vi "HexaboardCenterFinderLaserHoleAI.vi"() -> ()   [LabVIEW 2019]
uses:
  <vilib>/userDefined/High Color/IMAQdx.ctl
  <vilib>/Analysis/coordinate.llb/2D Cartesian Coordinate Rotation (Scalar).vi
  <vilib>/Utility/file.llb/Read Delimited Spreadsheet (DBL).vi
  Other Models/2010/Motion/AbortSingle.vi
  <vilib>/Analysis/NI_AALPro.lvlib
panel:
  out "error out":errorcluster
  out "CameraGcode":string
  out "Center_XYZU":string
  out "Image 2":T1(plugin-control)
  out "Image":T1(plugin-control)
  in  "YoffsetPos1":dbl=24.138
  in  "XoffsetPos1":dbl=6.964
  in  "ModuleName":string="T1"
  in  "StopJoyStick":bool
  out "CurrentImage":T1(plugin-control)
  in  "CoordFileIn":string="HB_LaserHoles.txt"
  out "UsedCoordinates":string
  in  "Position":enum16{"1", "2"}(ring)
  in  "Zone":enum16{"ZoneA", "ZoneB", "ZoneC", "ZoneD"}(ring)
  in  "InitialStepSize":dbl=0.05
  in  "AbortAutoFocus":bool
  in  "AutoFocus":bool=TRUE
  in  "VisibilityInCamera":enum16{"JoyStick", "AllVisible"}(ring)=enum."AllVisible"
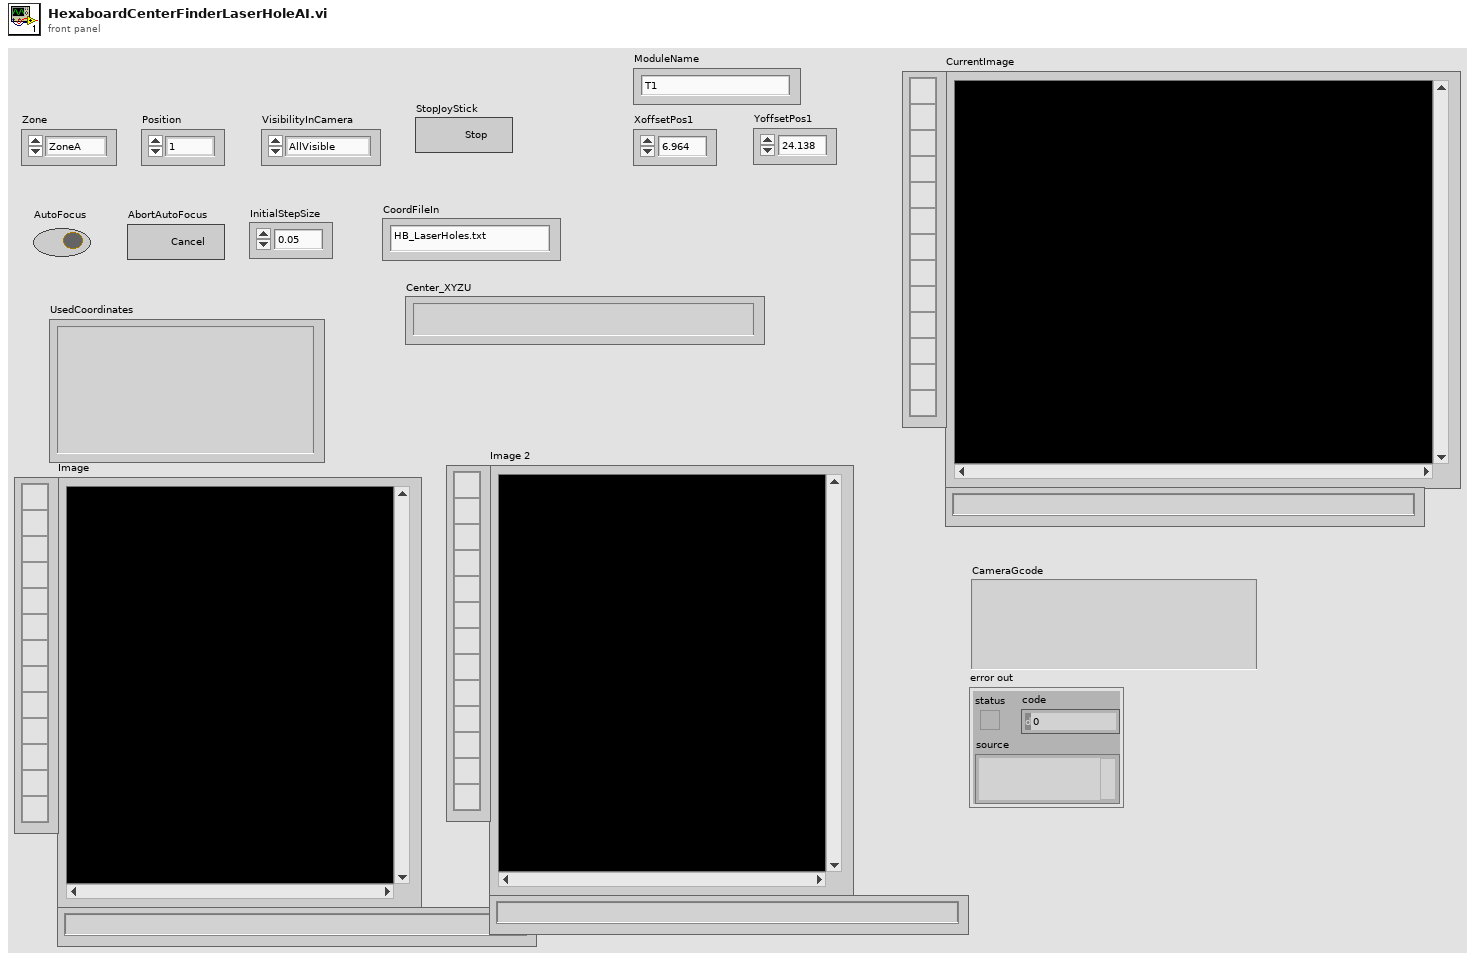
[diagram p1: front panel]
types:
  T1 = typedef "IMAQ Image.ctl" = refnum<image>
  T2 = typedef "Image Type" = u32
  T3 = typedef "IMAQdx.ctl" = refnum<k21>
  T4 = enum16{"Left Button", "Center Button", "Right Button", "Window Close"}
  T5 = enum16{"open", "replace", "create", "open or create", "replace or create", "replace or create with confirmation"}
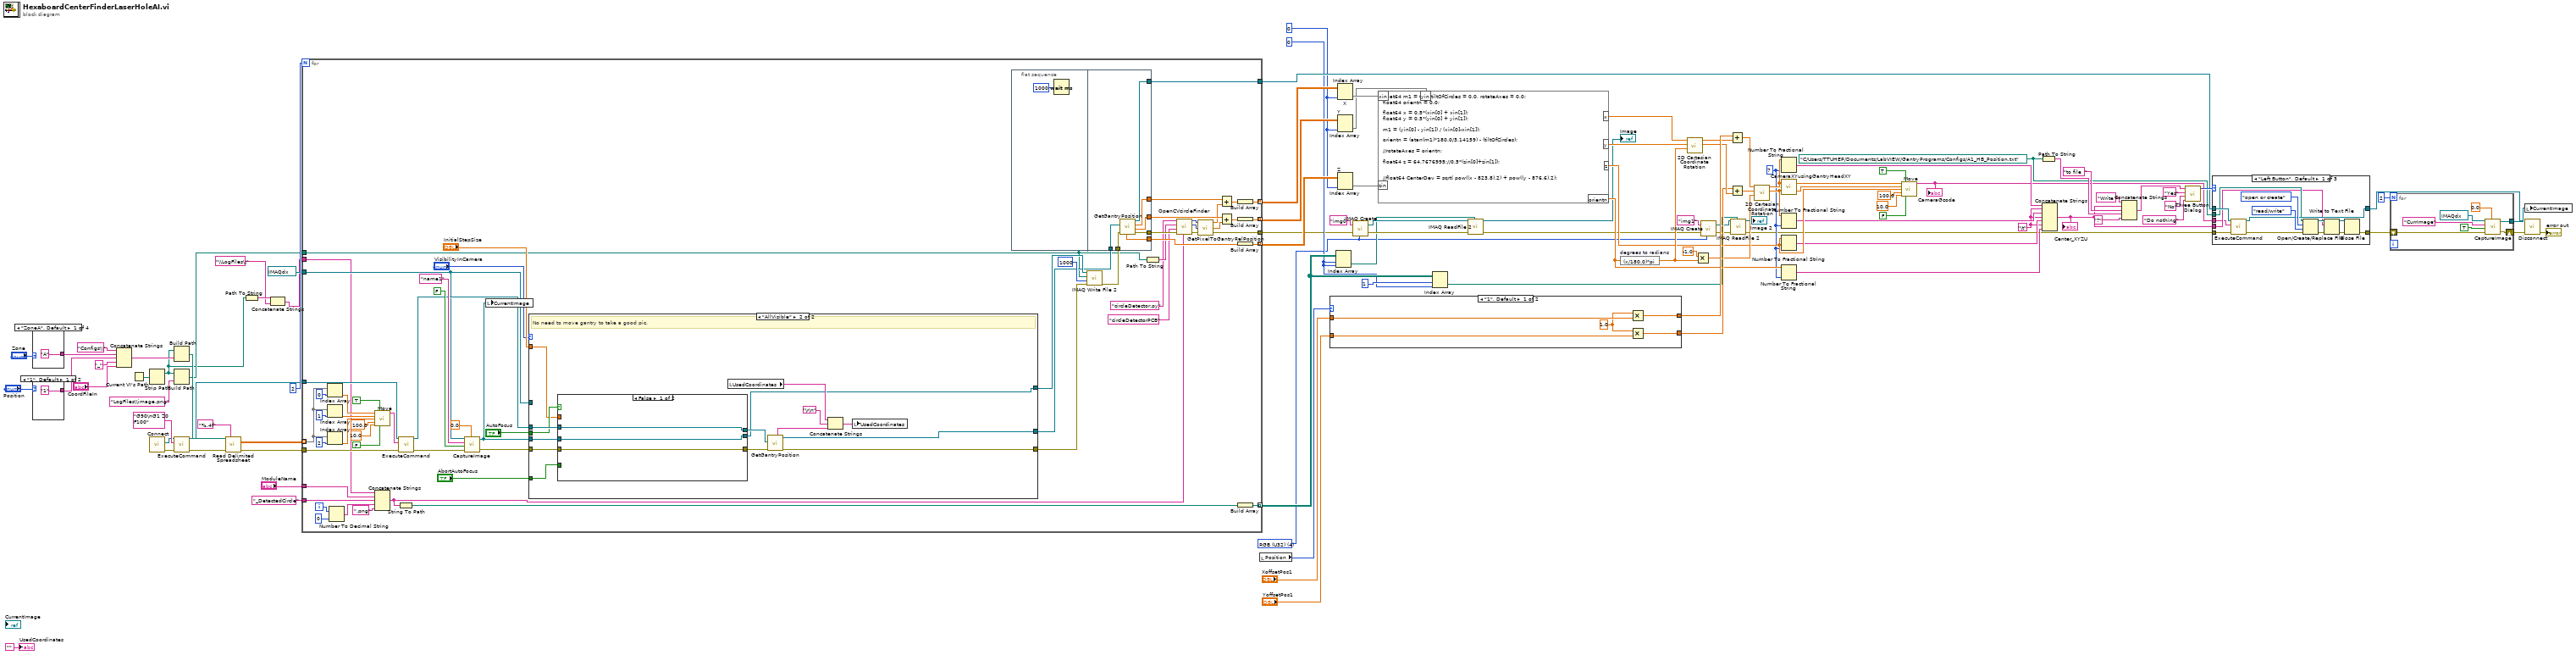
[diagram p0: block diagram]
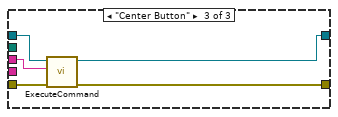
[diagram p3: hidden frame]
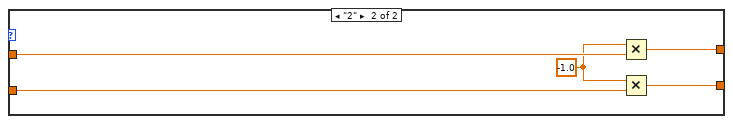
[diagram p4: hidden frame]
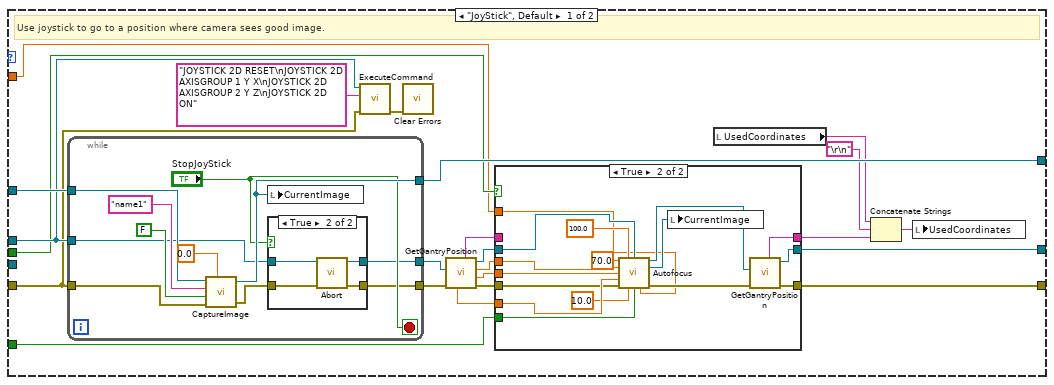
[diagram p5: hidden frame]
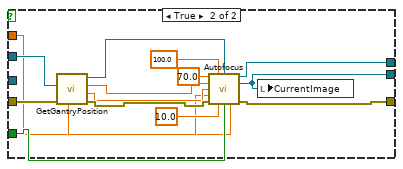
[diagram p8: hidden frame]
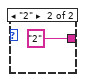
[diagram p9: hidden frame]
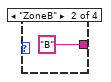
[diagram p10: hidden frame]
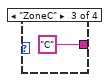
[diagram p11: hidden frame]
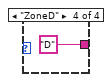
[diagram p12: hidden frame]
diagram:
  w14 = T2 4 items=["Grayscale (U8)", "Grayscale (I16)", "Grayscale (SGL)", "Complex (CSG)", "RGB (U32)", "HSL (U32)", "RGB (U64)", "Grayscale (U16)"] ("Image Type")
  w18 = 0 ("index")
  w44 = "\t"
  w45 = i16 7 ("precision (6)")
  w33 = path "C:/Users/TTUHEP/Documents/LabVIEW/GantryPrograms/Configs/A1_HB_Position.txt" ("OutFile")
  w24 = 0 ("disabled index (col)")
  n1 = case shown="\"ZoneA\", Default" "Zone" {
    tunnel: ["A" "B" "C" "D"] -> w99
    frame "ZoneA", Default {
    }
    frame "ZoneB" {
    }
    frame "ZoneC" {
    }
    frame "ZoneD" {
    }
  }
  n2 = case shown="\"1\", Default" "Position" {
    tunnel: ["1" "2"] -> w98
    frame "1", Default {
    }
    frame "2" {
    }
  }
  n3 = Concatenate Strings("Configs\\" ("string"), w99, w98, "_" ("string"), "CoordFileIn") -> (w93:string)
  n4 = Current VI's Path() -> (path=w96:path)
  n5 = Strip Path(path=w96) -> (stripped path=w4:path)  [unwired: 1 out]
  n6 = call "Connect.vi"() -> ("error out"=w90:errorcluster, "controller"=w91:refnum<k24>)  [unwired: 10 in]
  n7 = Build Path(base path=w4, name or relative path=w93) -> (appended path=w88:path)
  n8 = Build Path(base path=w4, name or relative path="LogFiles\\image.png") -> (appended path=w80:path)
  n9 = call "ExecuteCommand.vi"("error in (no error)"=w90, "Command Code"="G90\nG1 Z0 F100", "controller in"=w91) -> ("error out"=w87:errorcluster, "controller out"=w84:refnum<k24>)  [unwired: 6 in, 1 out]
  n10 = call-poly <vilib>:"Read Delimited Spreadsheet.vi"("file path (dialog if empty)"=w88, "format (%.3f)"="%.4f", "error in (no error)"=w87) -> ("all rows"=w86:dbl[][], "error out"=w83:errorcluster)  [unwired: 7 in, 4 out]
  n11 = Path To String(path=w4) -> (string=w3:string)
  n12 = Concatenate Strings(w3, "\\LogFiles\\") -> (w1:string)
  n13 = for {
    N: 2 -> [_]
    tunnel: w86 -> [w167] mode=indexing
    tunnel: w84 -> [w158]
    tunnel: w83 -> [w157]
    tunnel: T3 "cam1" ("Camera") -> [w149]
    tunnel: w80 -> [w116]
    tunnel: w1 -> [w137]
    tunnel: "ModuleName" -> [w136]
    tunnel: "_DetectedCircle" ("string") -> [w135]
    tunnel: [w129] -> w77 mode=indexing
    tunnel: [w128] -> w76 mode=indexing
    tunnel: [w126] -> w25 mode=indexing
    tunnel: [w125] -> w34
    tunnel: [w112] -> w8
    tunnel: [w111] -> w19 mode=indexing
    i -> [w134]
    n14 = Index Array(array=w167, index=0) -> (element=w166:dbl)
    n15 = Index Array(array=w167, index=1) -> (element=w165:dbl)
    n16 = Index Array(array=w167, index=2) -> (element=w164:dbl)
    n17 = Number To Decimal String(number=w134, width (-)=i16 0) -> (decimal integer string=w123:string)
    n18 = call "Move.vi"("X"=w166, "Absolute"=TRUE, "Y"=w165, "Z"=w164, "SpeedXY (mm/s)"=100.0, "SpeedZ (mm/s)"=10.0, "Move Z first"=FALSE) -> ("Position Gcode"=w159:string)  [unwired: 8 in]
    n19 = Concatenate Strings(w137, w136, w135, w123, ".png" ("string")) -> (w110:string)
    n20 = String To Path(string=w110) -> (path=w109:path)
    n21 = call "ExecuteCommand.vi"("error in (no error)"=w157, "Command Code"=w159, "controller in"=w158) -> ("error out"=w154:errorcluster, "controller out"=w150:refnum<k24>)  [unwired: 6 in, 1 out]
    n22 = call "CaptureImage.vi"("Camera"=w149, "Rotate (degrees)"=sgl 0.0, "ImageName"="name1", "Draw50MicroCircleAtCenter"=FALSE, "error in (no error)"=w154) -> ("Image"=w145:T1, "error out"=w148:errorcluster)  [unwired: 2 in]
    n23 = local write "CurrentImage"(w145) -> ()
    n24 = case shown="\"AllVisible\"" "VisibilityInCamera" {
      tunnel: w149 -> [w199 _]
      tunnel: w150 -> [w197 w250]
      tunnel: w148 -> [w195 w251]
      tunnel: [w198 w239] -> w143
      tunnel: [w182 w245] -> w140
      tunnel: [w183 w243] -> w142
      tunnel: "AbortAutoFocus" -> [w186 w248]
      tunnel: "AutoFocus" -> [w180 w249]
      tunnel: "InitialStepSize" -> [w179 w247]
      tunnel: w145 -> [_ w238]
      frame "JoyStick", Default {
        # "Use joystick to go to a position where camera sees good image."
        n25 = while {
          tunnel: w199 -> [w229]
          tunnel: [w226] -> w198
          tunnel: w197 -> [w225]
          tunnel: [w222] -> w193
          tunnel: [w221] -> w194
          tunnel: w195 -> [w220]
          stop <- "StopJoyStick" stop-if-true
          n26 = call "CaptureImage.vi"("Camera"=w229, "Rotate (degrees)"=sgl 0.0, "ImageName"="name1", "Draw50MicroCircleAtCenter"=FALSE, "error in (no error)"=w220) -> ("Image"=w226:T1, "error out"=w223:errorcluster)  [unwired: 2 in]
          n27 = local write "CurrentImage"(w226) -> ()
          n28 = case shown="True" "StopJoyStick" {
            tunnel: w225 -> [w232 w236]
            tunnel: w223 -> [w231 w235]
            tunnel: [w231 w234] -> w222
            tunnel: [w232 w233] -> w221
            frame False {
            }
            frame True {
              n29 = call-poly "Abort.vi"("error in (no error)"=w235, "controller in"=w236) -> ("error out"=w234:errorcluster, "controller out"=w233:refnum<k24>)  [unwired: 8 in]
            }
          }
        }
        n30 = call "ExecuteCommand.vi"("error in (no error)"=w195, "Command Code"="JOYSTICK 2D RESET\nJOYSTICK 2D AXISGROUP 1 Y X\nJOYSTICK 2D AXISGROUP 2 Y Z\nJOYSTICK 2D ON", "controller in"=w197) -> ("error out"=w196:errorcluster)  [unwired: 6 in, 2 out]
        n31 = call <vilib>:"Clear Errors.vi"("error in (no error)"=w196) -> ()  [unwired: 5 in, 2 out]
        n32 = call "GetGantryPosition.vi"("error in (no error)"=w193, "Controller In"=w194) -> ("error out"=w187:errorcluster, "Position Y"=w189:dbl, "Position X"=w190:dbl, "controller out"=w185:refnum<k24>, "Position_XYZ"=w181:string, "Position Z"=w188:dbl)  [unwired: 3 in, 1 out]
        n33 = case shown="True" w180 {
          tunnel: w190 -> [_ w219]
          tunnel: w189 -> [_ w218]
          tunnel: w188 -> [_ w217]
          tunnel: w187 -> [w203 w216]
          tunnel: w186 -> [_ w214]
          tunnel: w185 -> [w201 w213]
          tunnel: [w202 w209] -> w184
          tunnel: [w203 w208] -> w183
          tunnel: [w201 w207] -> w182
          tunnel: w181 -> [w202 _]
          tunnel: w179 -> [_ w205]
          frame False {
          }
          frame True {
            n34 = call "Autofocus.vi"("SafeMaxZ"=70.0, "SpeedXY (mm/s)"=100.0, "controller in"=w213, "X"=w219, "Y"=w218, "Z"=w217, "error in (no error)"=w216, "SpeedZ (mm/s)"=10.0, "AbortAutoFocus"=w214, "InitialStepSize"=w205) -> ("controller out"=w211:refnum<k24>, "Image"=w206:T1, "error out"=w210:errorcluster)  [unwired: 1 in, 2 out]
            n35 = local write "CurrentImage"(w206) -> ()
            n36 = call "GetGantryPosition.vi"("error in (no error)"=w210, "Controller In"=w211) -> ("error out"=w208:errorcluster, "controller out"=w207:refnum<k24>, "Position_XYZ"=w209:string)  [unwired: 3 in, 4 out]
          }
        }
        n37 = local read "UsedCoordinates"() -> (w191:string)
        n38 = Concatenate Strings(w191, "\r\n", w184) -> (w192:string)
        n39 = local write "UsedCoordinates"(w192) -> ()
      }
      frame "AllVisible" {
        # "No need to move gantry to take a good pic."
        n40 = case shown="False" w249 {
          tunnel: w248 -> [_ w268]
          tunnel: [w254 w265] -> w244
          tunnel: [w253 w266] -> w246
          tunnel: w251 -> [w254 w264]
          tunnel: w250 -> [w253 w263]
          tunnel: w247 -> [_ w257]
          tunnel: w238 -> [w252 _]
          tunnel: [w252 w256] -> w239
          frame False {
          }
          frame True {
            n41 = call "GetGantryPosition.vi"("error in (no error)"=w264, "Controller In"=w263) -> ("error out"=w262:errorcluster, "Position Y"=w261:dbl, "Position X"=w260:dbl, "controller out"=w259:refnum<k24>, "Position Z"=w258:dbl)  [unwired: 3 in, 2 out]
            n42 = call "Autofocus.vi"("SafeMaxZ"=70.0, "SpeedXY (mm/s)"=100.0, "controller in"=w259, "X"=w260, "Y"=w261, "Z"=w258, "error in (no error)"=w262, "SpeedZ (mm/s)"=10.0, "AbortAutoFocus"=w268, "InitialStepSize"=w257) -> ("controller out"=w266:refnum<k24>, "Image"=w256:T1, "error out"=w265:errorcluster)  [unwired: 1 in, 2 out]
            n43 = local write "CurrentImage"(w256) -> ()
          }
        }
        n44 = local read "UsedCoordinates"() -> (w241:string)
        n45 = call "GetGantryPosition.vi"("error in (no error)"=w244, "Controller In"=w246) -> ("error out"=w243:errorcluster, "controller out"=w245:refnum<k24>, "Position_XYZ"=w242:string)  [unwired: 3 in, 4 out]
        n46 = Concatenate Strings(w241, "\r\n", w242) -> (w240:string)
        n47 = local write "UsedCoordinates"(w240) -> ()
      }
    }
    n48 = flat-sequence {
      tunnel: w141 -> [w177]
      tunnel: w140 -> [w176]
      tunnel: [w175] -> w122
      tunnel: [w174] -> w139
      tunnel: [w173] -> w138
      tunnel: [w172] -> w127
      tunnel: [w171] -> w125
      frame #0 {
        n49 = Wait (ms)(milliseconds to wait=u32 1000) -> ()  [unwired: 1 out]
      }
      frame #1 {
        n50 = call "GetGantryPosition.vi"("error in (no error)"=w177, "Controller In"=w176) -> ("error out"=w175:errorcluster, "Position Y"=w173:dbl, "Position X"=w174:dbl, "controller out"=w171:refnum<k24>, "Position Z"=w172:dbl)  [unwired: 3 in, 2 out]
      }
    }
    n51 = call-poly "IMAQ Write File 2"("error in (no error)"=w142, "Image Quality"=u32 1000, "File Path"=w116, "Image"=w143) -> ("error out"=w141:errorcluster)  [unwired: 6 in, 1 out]
    n52 = Path To String(path=w116) -> (string=w120:string)
    n53 = call "OpenCVcircleFinder.vi"("OutFileName"=w110, "error in (no error)"=w122, "PyFunctionName"="circleDetectorPCB", "ImageFileName"=w120, "PythonFile"="circleDetector.py") -> ("error out"=w113:errorcluster, "CenterY0"=w115:u16, "CenterX0"=w114:u16)  [unwired: 1 in, 3 out]
    n54 = call "GetPixelToGantryRelPosition.vi"("error in (no error)"=w113, "PixelY"=w115, "PixelX"=w114) -> ("error out"=w112:errorcluster, "YmmRelGH"=w118:dbl, "XmmRelGH"=w117:dbl)
    n55 = Add(x=w139, y=w117) -> (x+y=w131:dbl)
    n56 = Add(x=w138, y=w118) -> (x+y=w130:dbl)
    n57 = Build Array(w131) -> (w129:dbl[])
    n58 = Build Array(w130) -> (w128:dbl[])
    n59 = Build Array(w127) -> (w126:dbl[])
    n60 = Build Array(w109) -> (w111:path[])
  }
  n61 = local read "Position"() -> (w71:enum16{"1", "2"})
  n62 = case shown="\"1\", Default" w71 {
    tunnel: "XoffsetPos1" -> [w274 w279]
    tunnel: "YoffsetPos1" -> [w272 w277]
    tunnel: [w271 w276] -> w68
    tunnel: [w270 w275] -> w65
    frame "1", Default {
      w273 = 1.0 ("x")
      n63 = Multiply(x=w273, y=w274) -> (x*y=w271:dbl)
      n64 = Multiply(x=w273, y=w272) -> (x*y=w270:dbl)
    }
    frame "2" {
      w278 = -1.0 ("x")
      n65 = Multiply(x=w278, y=w279) -> (x*y=w276:dbl)
      n66 = Multiply(x=w278, y=w277) -> (x*y=w275:dbl)
    }
  }
  n67 = Index Array(array=w19, index (row)=w18, index (col)=w18) -> (element=w17:path)
  n68 = Index Array "X"(array=w77, index (col)=w24) -> (element=w75:dbl[])  [unwired: 1 in]
  n69 = Index Array "Y"(array=w76, index (col)=w24) -> (element=w74:dbl[])  [unwired: 1 in]
  n70 = Index Array "Z"(array=w25, index (col)=w24) -> (element=w26:dbl[])  [unwired: 1 in]
  n71 = call "IMAQ Create"("Image Name"="img0", "Image Type"=w14, "error in (no error)"=w8) -> ("New Image"=w21:T1, "error out"=w20:errorcluster)  [unwired: 2 in]
  n72 = formula code="float64 m1 = 0.0, tiltOfCircles = 0.0, rotateAxes = 0.0;\nfloat64 orientn = 0.0;\n\nfloat64 x = 0.5*(xin[0] + xin[1]); \nfloat64 y = 0.5*(yin[0] + yin[1]);\n\nm1 = (yin[0] - yin[1]) / (xin[0]-xin[1]);\n\norientn = (atan(m1)*180.0/3.14159) - (tiltOfCircles);\n\n//rotateAxes = orientn;\n\nfloat64 z = 64.7676995;//0.5*(zin[0]+zin[1]);\n\n\n//float64 CenterDev = sqrt( pow((x - 823.8),2) + pow((y - 876.6),2);"("xin"=w75, "yin"=w74, "zin"=w26) -> ("orientn"=w46:dbl, "x"=w73:dbl, "y"=w72:dbl, "z"=w51:dbl)
  n73 = Index Array(array=w19, index (row)=1 ("index"), index (col)=w18) -> (element=w6:path)
  n74 = call "IMAQ ReadFile 2"("File Path"=w17, "error in (no error)"=w20, "Image"=w21) -> ("error out"=w13:errorcluster, "Image Out"=→"Image":T1)  [unwired: 4 in, 3 out]
  n75 = expression code="(x/180.0)*pi" "degrees to radians"(w46) -> (w61:dbl)
  n76 = call-poly <vilib>:"2D Cartesian Coordinate Rotation.vi"("theta"=w61, "y"=w72, "x"=w73) -> ("y out"=w66:dbl, "x out"=w67:dbl)  [unwired: 6 in, 1 out]
  n77 = Multiply(x=-1.0, y=w61) -> (x*y=w60:dbl)
  n78 = call "IMAQ Create"("Image Name"="img1", "Image Type"=w14, "error in (no error)"=w13) -> ("New Image"=w16:T1, "error out"=w15:errorcluster)  [unwired: 2 in]
  n79 = Add(x=w68, y=w67) -> (x+y=w64:dbl)
  n80 = Add(x=w65, y=w66) -> (x+y=w63:dbl)
  n81 = call "IMAQ ReadFile 2"("File Path"=w6, "error in (no error)"=w15, "Image"=w16) -> ("error out"=w7:errorcluster, "Image Out"=→"Image 2":T1)  [unwired: 4 in, 3 out]
  n82 = call-poly <vilib>:"2D Cartesian Coordinate Rotation.vi"("theta"=w60, "y"=w63, "x"=w64) -> ("y out"=w52:dbl, "x out"=w53:dbl)  [unwired: 6 in, 1 out]
  n83 = Number To Fractional String(number=w53, precision (6)=w45) -> (F-format string=w49:string)  [unwired: 2 in]
  n84 = call "CameraXYusingGantryHeadXY.vi"("GantryY"=w52, "GantryX"=w53) -> ("CamY"=w58:dbl, "CamX"=w59:dbl)
  n85 = Number To Fractional String(number=w52, precision (6)=w45) -> (F-format string=w48:string)  [unwired: 2 in]
  n86 = Number To Fractional String(number=w51, precision (6)=w45) -> (F-format string=w47:string)  [unwired: 2 in]
  n87 = Number To Fractional String(number=w46, precision (6)=w45) -> (F-format string=w43:string)  [unwired: 2 in]
  n88 = call "Move.vi"("X"=w59, "Absolute"=TRUE, "Y"=w58, "Z"=w51, "SpeedXY (mm/s)"=100.0, "SpeedZ (mm/s)"=10.0, "Move Z first"=FALSE) -> ("Position Gcode"=w31:string)  [unwired: 8 in]
  "CameraGcode" <- w31
  n89 = Path To String(path=w33) -> (string=w41:string)
  n90 = Concatenate Strings(w49, w44, w48, w44, w47, w44, w43) -> (w32:string)
  "Center_XYZU" <- w32
  n91 = Concatenate Strings("Write ", w32, "to file  ", w41, "?" ("string")) -> (w39:string)
  n92 = call <vilib>:"Three Button Dialog.vi"("Right Button Text (\"Cancel\")"="Do nothing" ("Right Button Text (\"Cancel\")"), "Center Button Text (\"No\")"="No" ("Center Button Text (\"No\")"), "Left Button Text (\"Yes\")"="Yes" ("Left Button Text (\"Yes\")"), "message"=w39) -> ("Which Button?"=w35:T4)  [unwired: 7 in]
  n93 = case shown="\"Left Button\", Default" w35 {
    tunnel: w34 -> [w283 w294 w297]
    tunnel: w7 -> [w284 w295 w300]
    tunnel: [w285 w295 w298] -> w30
    tunnel: [w289 w294 w299] -> w27
    tunnel: w33 -> [w282 _ _]
    tunnel: w32 -> [w281 _ _]
    tunnel: w31 -> [w280 _ w296]
    frame "Left Button", Default {
      n94 = call "ExecuteCommand.vi"("error in (no error)"=w284, "Command Code"=w280, "controller in"=w283) -> ("error out"=w286:errorcluster, "controller out"=w289:refnum<k24>)  [unwired: 6 in, 1 out]
      n95 = Open/Create/Replace File(file path (use dialog)=w282, error in=w286, operation (0:open)=T5."open or create", access (0:read/write)=enum16{"read/write", "read-only", "write-only"}."read/write") -> (refnum out=w288:refnum<file>, error out=w287:errorcluster)  [unwired: 2 in, 1 out]
      n96 = Write to Text File(file (use dialog)=w288, text=w281, error in=w287) -> (refnum out=w290:refnum<file>, error out=w291:errorcluster)  [unwired: 1 in, 1 out]
      n97 = Close File(refnum=w290, error in=w291) -> (error out=w285:errorcluster)  [unwired: 1 out]
    }
    frame "Right Button" {
    }
    frame "Center Button" {
      n98 = call "ExecuteCommand.vi"("error in (no error)"=w300, "Command Code"=w296, "controller in"=w297) -> ("error out"=w298:errorcluster, "controller out"=w299:refnum<k24>)  [unwired: 6 in, 1 out]
    }
  }
  n99 = for {
    N: 2 -> [_]
    tunnel: [w303] -> w29
    shift-right: [w301] -> w28
    shift-left: w30 -> [w304]
    n100 = call "CaptureImage.vi"("Camera"=T3 "cam1", "Rotate (degrees)"=sgl 0.0, "ImageName"="CurrImage", "Draw50MicroCircleAtCenter"=TRUE, "error in (no error)"=w304) -> ("Image"=w303:T1, "error out"=w301:errorcluster)  [unwired: 2 in]
  }
  n101 = local write "CurrentImage"(w29) -> ()
  n102 = call "Disconnect.vi"("error in (no error)"=w28, "controller"=w27) -> ("error out"=→"error out":errorcluster)  [unwired: 9 in]
  "UsedCoordinates" <- ""
